vi "Byte Array to Hex String.vi"(11 "Byte Array":u8[](array[numeric])) -> (3 "Hex String":string)   [LabVIEW 2021, in "dotNET Crypto Utility.lvlib"]
doc: "Converts the byte array to a lowercase hex string representation."
uses:
  dotNET Crypto Utility.lvlib
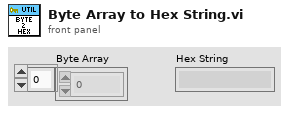
[diagram p1: front panel]
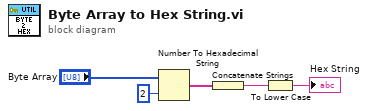
[diagram p0: block diagram]
diagram:
  n1 = Number To Hexadecimal String(1:i16 2 ("width (-)"), 2:"Byte Array") -> (0:w3:string[])
  n2 = Concatenate Strings(w3) -> (w2:string)
  n3 = To Lower Case(string=w2) -> (all lower case string=→"Hex String":string)
